vi "ZMQ.TestLauncher.REQ.vi"() -> ()   [LabVIEW 2016, in "ZMQ_SMO.lvclass"]
uses:
  ZMQ_SMO.lvclass
  <vilib>/JKI/JKI SMO/SMO/Typedefs/SMOState --Enum.ctl
  Typedefs/PublicEvents--ZMQ.ZMQ_PublicEvent.ctl
  C:/Program Files (x86)/National Instruments/LabVIEW 2016/vi.lib/JKI/JKI SMO/SMO/SMO.lvclass
  Typedefs/ZMQ Config.ctl
  <vilib>/addons/zeromq/socket_type.ctl
  ZMQ_SMO.lvclass/ZMQ_SMO.ctl
  <vilib>/JKI/JKI SMO/SMO/SMO.lvclass
  <vilib>/addons/zeromq/zeromq.lvlib
panel:
  in  "send message":bool
  out "message received":T1
  in  "messages to send":string[](array[string])
  out "SMO State":T2
  out "error out":errorcluster
  in  "Stop":bool
  # "REQ SMO Test Launcher"
  # "For instructions on how to use the JKI State Machine Objects, examples and video tutorials, visit:\nhttp://jki.net/state-machine-objects/\n\nJKI State Machine Objects™\nhttp://jki.net/state-machine-objects/\nCopyright (C) 2005-2015, JKI <info@jki.net>\nALL RIGHTS RESERVED"
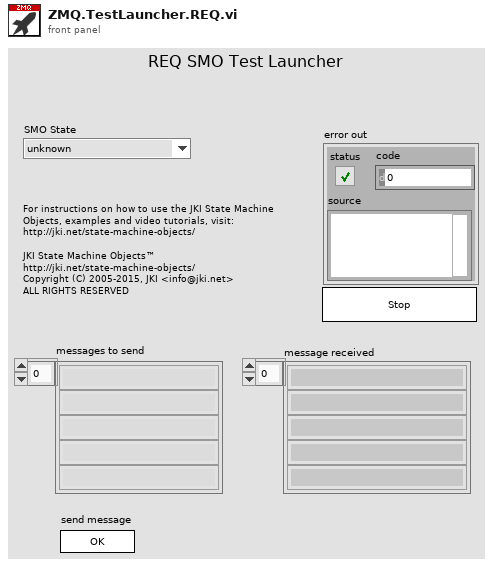
[diagram p1: front panel]
types:
  T1 = typedef "ZMQ_SMO.lvclass/PublicEvents--ZMQ.ZMQ_PublicEvent.ctl" = string[]
  T2 = typedef "SMO.lvclass/SMOState --Enum.ctl" = enum16{"unknown", "Created", "Started", "Stopped"}
  T3 = typedef "ZMQ_SMO.lvclass/ZMQ Config.ctl" = cluster{"socket type":T4, "endpoint":string, "filter":string}
  T4 = typedef "zeromq.lvlib/socket_type.ctl" = enum8{"ZMQ_PAIR", "ZMQ_PUB", "ZMQ_SUB", "ZMQ_REQ", "ZMQ_REP", "ZMQ_DEALER", "ZMQ_ROUTER", "ZMQ_PULL", "ZMQ_PUSH", "ZMQ_XPUB", "ZMQ_XSUB"}
  T5 = typedef "SMO.lvclass/Public Events.ctl" = cluster{"Error":refnum<user-event>, "State":refnum<user-event>, "Reserve State":refnum<user-event>}
  T6 = typedef "ZMQ_SMO.lvclass/PublicEvents--Cluster.ctl" = cluster{"ZMQ_message":refnum<user-event>}
  T7 = cluster{"Event Registration Refnum":refnum<event-registration>}
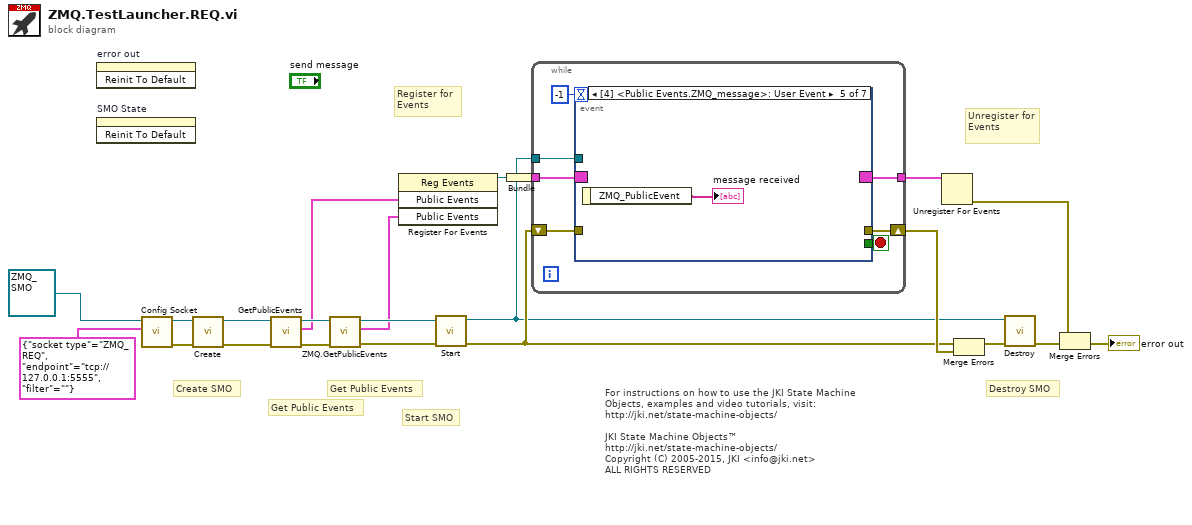
[diagram p0: block diagram]
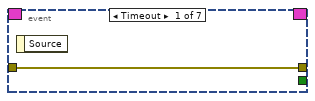
[diagram p2: hidden frame]
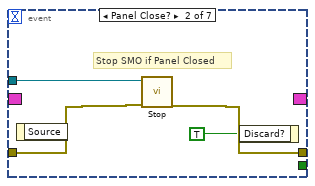
[diagram p3: hidden frame]
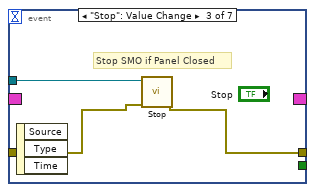
[diagram p4: hidden frame]
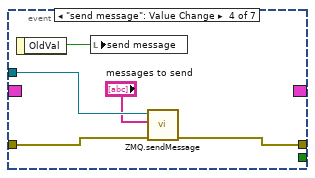
[diagram p5: hidden frame]
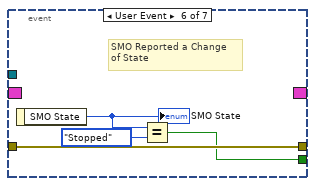
[diagram p6: hidden frame]
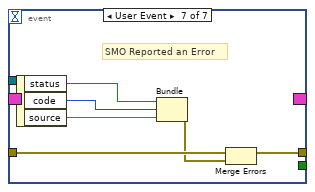
[diagram p7: hidden frame]
diagram:
  # "Get Public Events"
  # "For instructions on how to use the JKI State Machine Objects, examples and video tutorials, visit:\nhttp://jki.net/state-machine-objects/\n\nJKI State Machine Objects™\nhttp://jki.net/state-machine-objects/\nCopyright (C) 2005-2015, JKI <info@jki.net>\nALL RIGHTS RESERVED"
  # "Get Public Events"
  # "Start SMO"
  # "Destroy SMO"
  # "Create SMO"
  # "Unregister for Events"
  # "Register for Events"
  n1 = invoke on="error out" class="Clust (strict)" method="Reinit To Default"() -> ()  [unwired: 3 in, 3 out]
  n2 = invoke on="SMO State" class="Enum (strict)" method="Reinit To Default"() -> ()  [unwired: 3 in, 3 out]
  n3 = call "Config Socket.vi"("Socket Config"=T3 {"socket type"=enum."ZMQ_REQ", "endpoint"="tcp://127.0.0.1:5555", "filter"=""}, "ZMQ in"=refnum<class "ZMQ_SMO.lvclass"> refnum ("SMO.Template.lvclass")) -> ("error out"=w7:errorcluster, "ZMQ out"=w8:refnum<class "ZMQ_SMO.lvclass">)  [unwired: 8 in]
  n4 = call <vilib>:"Create.vi"("error in (no error)"=w7, "SMO"=w8) -> ("error out"=w13:errorcluster, "SMO out"=w14:refnum<class "ZMQ_SMO.lvclass">)  [unwired: 7 in, 1 out]
  n5 = call <vilib>:"GetPublicEvents.vi"("error in (no error)"=w13, "SMO"=w14) -> ("error out"=w4:errorcluster, "Public Events"=w2:T5, "SMO out"=w5:refnum<class "ZMQ_SMO.lvclass">)  [unwired: 7 in]
  n6 = call "ZMQ.GetPublicEvents.vi"("error in (no error)"=w4, "ZMQ"=w5) -> ("error out"=w11:errorcluster, "Public Events"=w3:T6, "ZMQ out"=w12:refnum<class "ZMQ_SMO.lvclass">)  [unwired: 7 in]
  n7 = register-events(w2, w3) -> (reference out=w6:refnum<event-registration>)  [unwired: 2 in, 1 out]
  n8 = call <vilib>:"Start.vi"("error in (no error)"=w11, "SMO"=w12) -> ("error out"=w16:errorcluster, "SMO out"=w10:refnum<class "ZMQ_SMO.lvclass">)  [unwired: 8 in]
  n9 = Bundle("Event Registration Refnum"=w6) -> (w21:T7)  [unwired: 1 in]
  n10 = while {
    shift-right: [w28] -> w20
    shift-left: w16 -> [w27]
    tunnel: w21 -> [w26]
    tunnel: [w25] -> w22
    tunnel: w10 -> [w24]
    stop <- w29 stop-if-true
    n11 = event shown="[4] <Public Events.ZMQ_message>: User Event" {
      selector: w26 -> [_ _ _ _ _ _ _]
      dyn-events: [_ _ _ _ _ _ _] -> w25
      timeout: -1 -> [_ _ _ _ _ _ _]
      tunnel: [_ _ _ _ _ w44 _] -> w29
      tunnel: w24 -> [_ w34 w37 w42 _ _ _]
      tunnel: [w30 w33 w36 w40 _ w47 w51] -> w28
      tunnel: w27 -> [w30 w32 w35 w41 _ w47 w49]
      event Timeout {
        n12 = event-data() -> ()  [unwired: 1 in, 1 out]
      }
      event Panel Close? {
        # "Stop SMO if Panel Closed"
        n13 = event-data() -> ()  [unwired: 1 in, 1 out]
        n14 = call <vilib>:"Stop.vi"("error in (no error)"=w32, "SMO"=w34) -> ("error out"=w33:errorcluster)  [unwired: 8 in, 1 out]
        n15 = event-data("Discard?"=TRUE ("OK")) -> ()  [unwired: 1 in, 1 out]
      }
      event "Stop": Value Change {
        # "Stop SMO if Panel Closed"
        n16 = event-data() -> ()  [unwired: 1 in, 3 out]
        n17 = call <vilib>:"Stop.vi"("error in (no error)"=w35, "SMO"=w37) -> ("error out"=w36:errorcluster)  [unwired: 8 in, 1 out]
      }
      event "send message": Value Change {
        n18 = event-data() -> ("OldVal"=w38:bool)  [unwired: 1 in]
        n19 = local write "send message"(w38) -> ()
        n20 = call "ZMQ.sendMessage.vi"("error in (no error)"=w41, "message"="messages to send", "ZMQ"=w42) -> ("error out"=w40:errorcluster)  [unwired: 7 in, 1 out]
      }
      event User Event {
        n21 = event-data() -> ("ZMQ_PublicEvent"=→"message received":T1)  [unwired: 1 in]
      }
      event User Event {
        # "SMO Reported a Change\nof State"
        n22 = event-data() -> ("SMO State"=w46:T2)  [unwired: 1 in]
        "SMO State" <- w46
        n23 = Equal?(x=w46, y=SMOState_--Enum."Stopped") -> (x = y?=w44:bool)
      }
      event User Event {
        # "SMO Reported an Error"
        n24 = event-data() -> ("status"=w50:bool, "code"=w53:i32, "source"=w52:string)  [unwired: 1 in]
        n25 = Bundle("status"=w50, "code"=w53, "source"=w52) -> (w48:errorcluster)  [unwired: 1 in]
        n26 = Merge Errors(w49, w48) -> (w51:errorcluster)
      }
    }
  }
  n27 = Unregister For Events(event registration refnum=w22) -> (error out=w19:errorcluster)  [unwired: 1 in]
  n28 = Merge Errors(w16, w20) -> (w15:errorcluster)
  n29 = call <vilib>:"Destroy.vi"("error in (no error)"=w15, "SMO"=w10) -> ("error out"=w17:errorcluster)  [unwired: 9 in]
  n30 = Merge Errors(w19, w17) -> (→"error out":errorcluster)
